vi "New Data Available.vi"(5 "Component ID":u8, 7 "FPGA Interface":refnum<class "FPGA Interface.lvclass">, 8 "error in (no error)":errorcluster, 10 "Rx SubAddress (1-30)":u16, 11 "Remote Terminal in":refnum<class "Remote Terminal.lvclass">) -> (0 "error out":errorcluster, 2 "New Data Available?":bool)   [LabVIEW 2020, in "BCI-1553 API.lvlib" / "Remote Terminal.lvclass"]
doc: "Checks IC memory to determine if a receive subaddress has received any data. This flag will latch high after the first time the subaddress receives data. Call the 'Clear Data Available Flag' method to reset the flag."
uses:
  Remote Terminal.lvclass
  Dependencies/FPGA Interface/FPGA Interface.lvclass
  Remote Terminal.lvclass/Remote Terminal.ctl
panel:
  out "debug":u16 format="%04x"
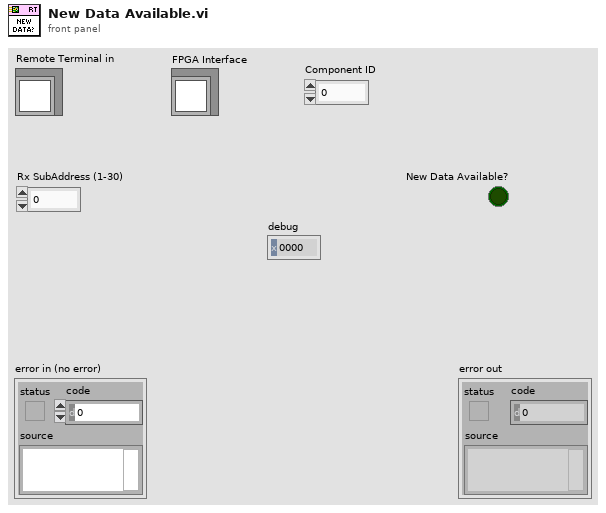
[diagram p1: front panel]
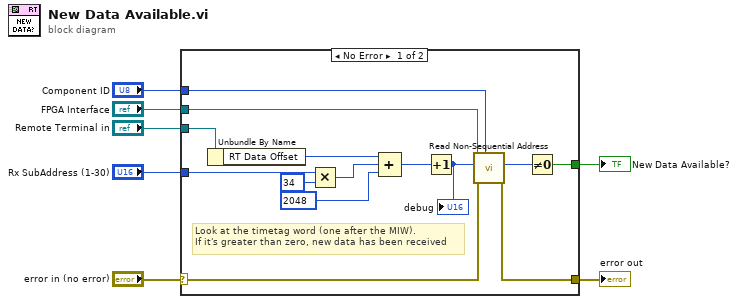
[diagram p0: block diagram]
diagram:
  n1 = case shown="No Error" "error in (no error)" {
    selector: "error in (no error)" -> [w13 w22]
    tunnel: [w12 w22] -> w6
    tunnel: "Remote Terminal in" -> [w15 _]
    tunnel: "Rx SubAddress (1-30)" -> [w14 _]
    tunnel: "FPGA Interface" -> [w10 _]
    tunnel: "Component ID" -> [w11 _]
    tunnel: [w9 _] -> w1
    frame No Error {
      # "Look at the timetag word (one after the MIW).\nIf it's greater than zero, new data has been received"
      n2 = Unbundle By Name(w15) -> ("RT Data Offset"=w18:u16)
      n3 = Multiply(x=w14, y=u16 34 ("Address")) -> (x*y=w17:u16)
      n4 = Compound Arithmetic op=ADD(w18, w17, u16 2048 ("Address")) -> (w19:u16)
      n5 = Increment(x=w19) -> (x+1=w20:u16)
      "debug" <- w20
      n6 = call-dynamic "Read Non-Sequential Address.vi"("Target IC (1-8)"=w11, "error in (no error)"=w13, "Address"=w20, "FPGA Interface in"=w10) -> ("error out"=w12:errorcluster, "Data"=w21:u16)  [unwired: 6 in]
      n7 = Not Equal To 0?(x=w21) -> (x != 0?=w9:bool)
    }
    frame Error {
    }
  }
  "error out" <- w6
  "New Data Available?" <- w1
